vi "Read Active.vi"(8 "error in (no error)":errorcluster, 11 "Droid in":refnum<class "Droid.lvclass">) -> (0 "error out":errorcluster, 2 "Active":bool, 3 "Droid out":refnum<class "Droid.lvclass">)   [LabVIEW 2021, in "Droid.lvclass"]
uses:
  Droid.lvclass
  Droid.lvclass/Droid.ctl
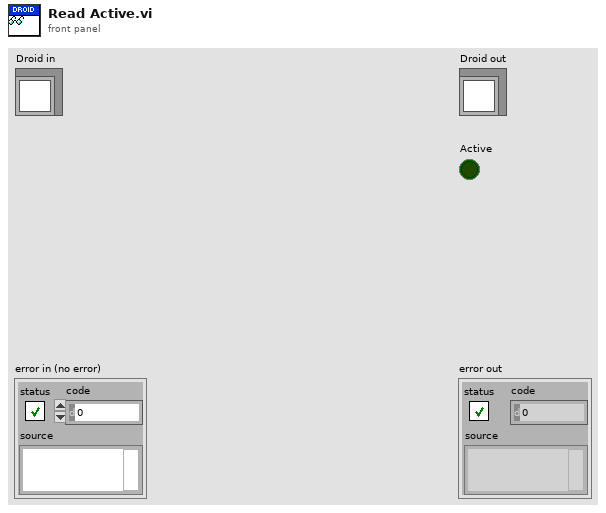
[diagram p1: front panel]
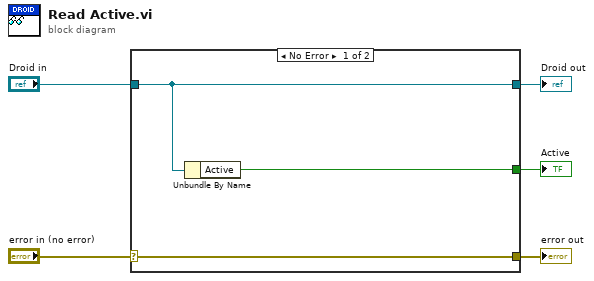
[diagram p0: block diagram]
diagram:
  n1 = case shown="No Error" "error in (no error)" {
    selector: "error in (no error)" -> [w8 w9]
    tunnel: [w8 w9] -> w4
    tunnel: [w7 w10] -> w2
    tunnel: "Droid in" -> [w7 w10]
    tunnel: [w6 _] -> w1
    frame No Error {
      n2 = Unbundle By Name(w7) -> ("Active"=w6:bool)
    }
    frame Error {
    }
  }
  "error out" <- w4
  "Droid out" <- w2
  "Active" <- w1
